vi "Simple Safe Move.vi"(7 "overwrite (F)":bool, 8 "error IO":errorcluster, 9 "Timeout (in 10 ms increments)":u32=100, 10 "Destination":path, 11 "Source File path":path) -> (0 "Erro Out":errorcluster, 3 "new path":path)   [LabVIEW 2017, in "G3_Build Process File Utilities.lvlib"]
doc: "Copys a file or directory to the specified destination and waits until the destination size equals the source size. \n\nTo Copy a file to a directory\nNo Rename: \\Source\\File.txt -> \\destination\nRename: \\Source\\File.txt-> \\destination\\NewFileName.txt\n\nTo copy a directory to a new directory:\nCopy source directroy into destination: \\Source -> \\Destination\nWARNING: this creates a sub directory at Destination called \"Source\" so that you know have Destination\\Source\\contents"
uses:
  G3_Build Process File Utilities.lvlib
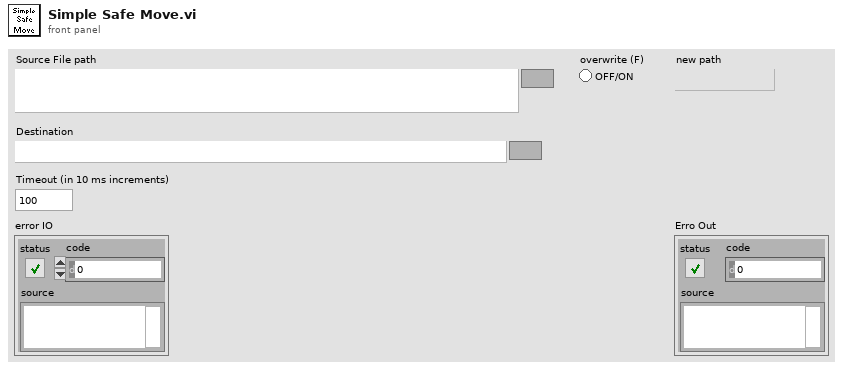
[diagram p1: front panel]
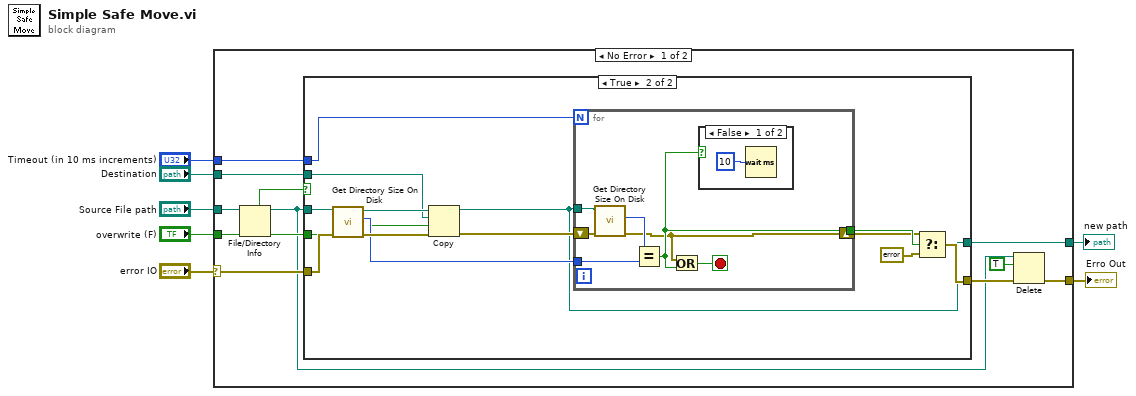
[diagram p0: block diagram]
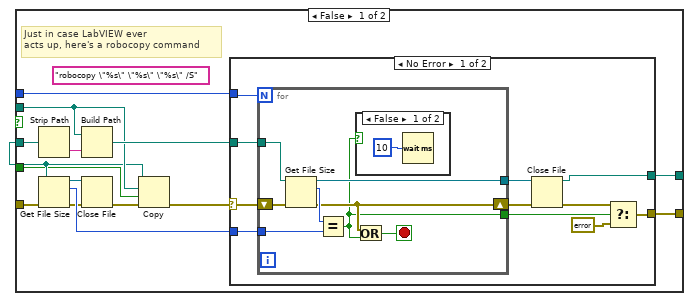
[diagram p2: hidden frame]
diagram:
  n1 = case shown="No Error" "error IO" {
    selector: "error IO" -> [w18 w76]
    tunnel: "Destination" -> [w17 _]
    tunnel: "Source File path" -> [w11 _]
    tunnel: [w16 w76] -> w4
    tunnel: "Timeout (in 10 ms increments)" -> [w14 _]
    tunnel: "overwrite (F)" -> [w13 _]
    tunnel: [w12 _] -> w1
    frame No Error {
      n2 = File/Directory Info(path=w11) -> (path out=w10:path, directory=w9:bool)  [unwired: 1 in, 5 out]
      n3 = case shown="True" w9 {
        tunnel: w18 -> [w31 w66]
        tunnel: w17 -> [w26 w64]
        tunnel: w10 -> [w23 w67]
        tunnel: [w22 w56] -> w15
        tunnel: w14 -> [w21 w61]
        tunnel: w13 -> [w20 w54]
        tunnel: [w19 w55] -> w12
        frame False {
          (unwired) "robocopy \"%s\" \"%s\" \"%s\" /S" ("command line")
          # "Just in case LabVIEW ever \nacts up, here's a robocopy command"
          n4 = Strip Path(path=w23) -> (name=w28:string)  [unwired: 1 out]
          n5 = Get File Size(file=w23, error in=w31) -> (refnum out=w29:refnum<file>, size (in bytes)=w32:i64, 0:w30:errorcluster)
          n6 = Build Path(base path=w26, name or relative path=w28) -> (appended path=w27:path)
          n7 = Close File(refnum=w29, error in=w30) -> (error out=w24:errorcluster)  [unwired: 1 out]
          n8 = Copy(8:w24, 9:w20, 10:w26, 11:w23) -> (0:w25:errorcluster)  [unwired: 1 in, 2 out]
          n9 = case shown="No Error" w25 {
            selector: w25 -> [w42 w53]
            tunnel: w27 -> [w34 _]
            tunnel: w32 -> [w43 _]
            tunnel: [w38 w53] -> w22
            tunnel: w21 -> [w35 _]
            tunnel: [w33 _] -> w19
            frame No Error {
              n10 = for {
                N: w35 -> [_]
                tunnel: w34 -> [w50]
                tunnel: [w49] -> w37
                tunnel: w43 -> [w47]
                shift-right: [w46] -> w36
                shift-left: w42 -> [w51]
                tunnel: [w45] -> w41
                stop <- w44 stop-if-true
                n11 = Get File Size(file=w50, error in=w51) -> (refnum out=w49:refnum<file>, size (in bytes)=w48:i64, 0:w46:errorcluster)
                n12 = Equal?(x=w48, y=w47) -> (x = y?=w45:bool)
                n13 = case shown="False" w45 {
                  frame False {
                    n14 = Wait (ms)(milliseconds to wait=u32 10) -> ()  [unwired: 1 out]
                  }
                  frame True {
                  }
                }
                n15 = Or(x=w46, y=w45) -> (x .or. y?=w44:bool)
              }
              n16 = Close File(refnum=w37, error in=w36) -> (path=w33:path, error out=w39:errorcluster)
              n17 = Select(t=w39, s=w41, f=errorcluster {"status"=TRUE, "code"=0, "source"="Destination file size did not equaly source file size by the specified timeout."}) -> (s? t:f=w38:errorcluster)
            }
            frame Error {
            }
          }
        }
        frame True {
          n18 = call "Get Directory Size On Disk.vi"("error in"=w66, "Path"=w67) -> ("error out"=w63:errorcluster, "Bytes"=w62:i32, "dup Path"=w65:path)  [unwired: 7 in]
          n19 = Copy(8:w63, 9:w54, 10:w64, 11:w65) -> (0:w58:errorcluster, 3:w55:path)  [unwired: 1 in, 1 out]
          n20 = for {
            N: w61 -> [_]
            tunnel: w62 -> [w74]
            shift-right: [w69] -> w57
            shift-left: w58 -> [w70]
            tunnel: [w73] -> w59
            tunnel: w55 -> [w68]
            stop <- w72 stop-if-true
            n21 = call "Get Directory Size On Disk.vi"("error in"=w70, "Path"=w68) -> ("error out"=w69:errorcluster, "Bytes"=w71:i32)  [unwired: 7 in, 1 out]
            n22 = Equal?(x=w71, y=w74) -> (x = y?=w73:bool)
            n23 = Or(x=w69, y=w73) -> (x .or. y?=w72:bool)
            n24 = case shown="False" w73 {
              frame False {
                n25 = Wait (ms)(milliseconds to wait=u32 10) -> ()  [unwired: 1 out]
              }
              frame True {
              }
            }
          }
          n26 = Select(t=w57, s=w59, f=errorcluster {"status"=TRUE, "code"=0, "source"="Destination file size did not equaly source file size by the specified timeout."}) -> (s? t:f=w56:errorcluster)
        }
      }
      n27 = Delete(path (use dialog)=w10, entire hierarchy (F)=TRUE, error in=w15) -> (error out=w16:errorcluster)  [unwired: 2 in, 2 out]
    }
    frame Error {
    }
  }
  "Erro Out" <- w4
  "new path" <- w1
